vi "decodeFloat64.vi"(8 "error in (no error)":errorcluster, 10 "ByteArray":u8[](array[numeric]) format="%.0x") -> (0 "error out":errorcluster, 1 "Float":dbl, 2 "variant":variant, 3 "RemainingBytes":u8[](array[numeric]), 5 "Type":string)   [LabVIEW 2016, in "MsgPack.lvlib"]
uses:
  MsgPack.lvlib
  <vilib>/Utility/error.llb/Error Cluster From Error Code.vi
  <vilib>/ErrorRing/Error Ring.xnode
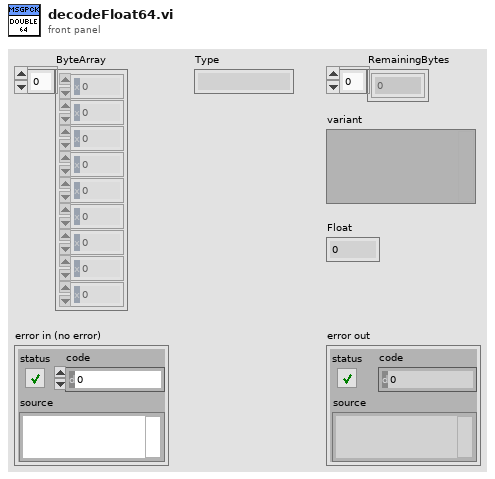
[diagram p1: front panel]
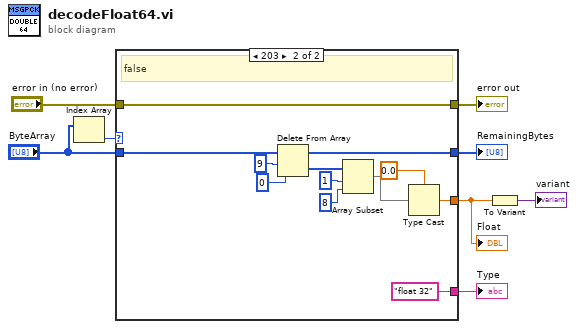
[diagram p0: block diagram]
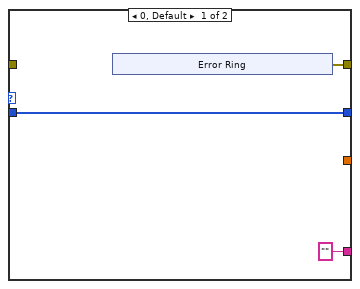
[diagram p2: hidden frame]
diagram:
  n1 = Index Array(array="ByteArray") -> (element=w5:u8)  [unwired: 1 in]
  n2 = case shown="203" w5 {
    tunnel: [w10 w28] -> w7
    tunnel: "error in (no error)" -> [_ w28]
    tunnel: ["" "float 32"] -> w4
    tunnel: "ByteArray" -> [w9 w21]
    tunnel: [_ w23] -> w3
    tunnel: [w9 w19] -> w1
    frame 0, Default {
      n3 = xnode "Error Ring"() -> ("error out"=w10:errorcluster)
    }
    frame 203 {
      # "false"
      n4 = Delete From Array(array=w21, length=9, index=0) -> (deleted portion=w18:u8[], array with subset deleted=w19:u8[])
      n5 = Array Subset(array=w18, index=1, length=8) -> (w24:u8[])
      n6 = Type Cast(type=0.0 ("Float"), x=w24) -> (*(type *) &x=w23:dbl)
    }
  }
  "error out" <- w7
  "Type" <- w4
  "Float" <- w3
  "RemainingBytes" <- w1
  n7 = To Variant(anything=w3) -> (Variant=→"variant":variant)
